vi "main.vi"() -> ()   [LabVIEW 2017]
panel:
  in  "Stop Button":bool
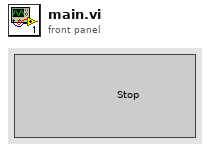
[diagram p1: front panel]
types:
  T1 = typedef "LVPositionTypeDef.ctl" = cluster{"Left":i32, "Top":i32}
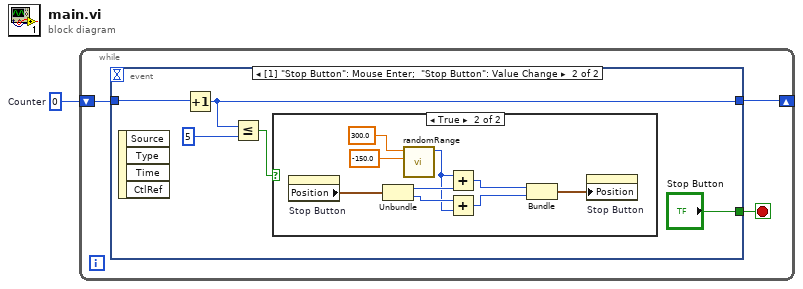
[diagram p0: block diagram]
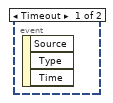
[diagram p2: hidden frame]
diagram:
  w1 = 0  # Counter
  n1 = while {
    shift-right: [w3] -> _
    shift-left: w1 -> [w4]
    stop <- w2 stop-if-true
    n2 = event shown="[1] \"Stop Button\": Mouse Enter;  \"Stop Button\": Value Change" {
      selector: _ -> [_ _]
      dyn-events: _ -> [_ _]
      timeout: _ -> [_ _]
      tunnel: w4 -> [_ w9]
      tunnel: [_ w7] -> w3
      tunnel: [_ "Stop Button"] -> w2
      event Timeout {
        n3 = event-data() -> ()  [unwired: 1 in, 3 out]
      }
      event "Stop Button": Mouse Enter; "Stop Button": Value Change {
        n4 = event-data() -> ()  [unwired: 1 in, 4 out]
        n5 = Increment(x=w9) -> (x+1=w7:i32)
        n6 = Less Or Equal?(x=w7, y=5) -> (x <= y?=w8:bool)
        n7 = case shown="True" w8 {
          frame False {
          }
          frame True {
            n8 = property on="Stop Button" class="Bool"() -> ("Position"=w11:T1)  [unwired: 2 in, 2 out]
            n9 = Unbundle(w11) -> ("Left"=w16:i32, "Top"=w15:i32)
            n10 = call "randomRange.vi"("Minimum value"=-150.0, "Range"=300.0) -> ("Random"=w14:i32)  [unwired: 9 in]
            n11 = Add(x=w14, y=w16) -> (x+y=w12:i32)
            n12 = Add(x=w15, y=w14) -> (x+y=w13:i32)
            n13 = Bundle(w12, w13) -> (w10:cluster{i32, i32})  [unwired: 1 in]
            n14 = property on="Stop Button" class="Bool"("Position"=w10) -> ()  [unwired: 2 in, 2 out]
          }
        }
      }
    }
  }
